vi "Replace Outside Typedef Control.vi"(6 "Dependent VIs":path[](array[path]), 8 "error in (no error)":errorcluster, 9 "Shared directory":path, 10 "Non-Library VI[]":string[](array[string]), 11 "Measurement Directory":path) -> (0 "error out":errorcluster)   [LabVIEW 2021, in "Multiple Converter.lvlib"]
uses:
  Multiple Converter.lvlib
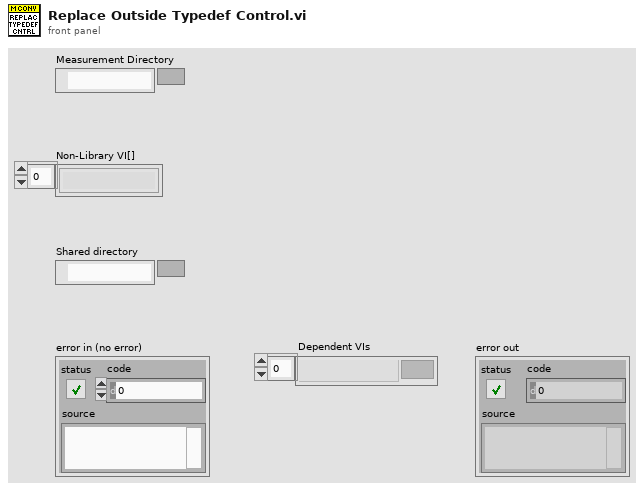
[diagram p1: front panel]
types:
  T1 = enum32{"not a typedef", "typedef", "strict typedef", "class private data"}
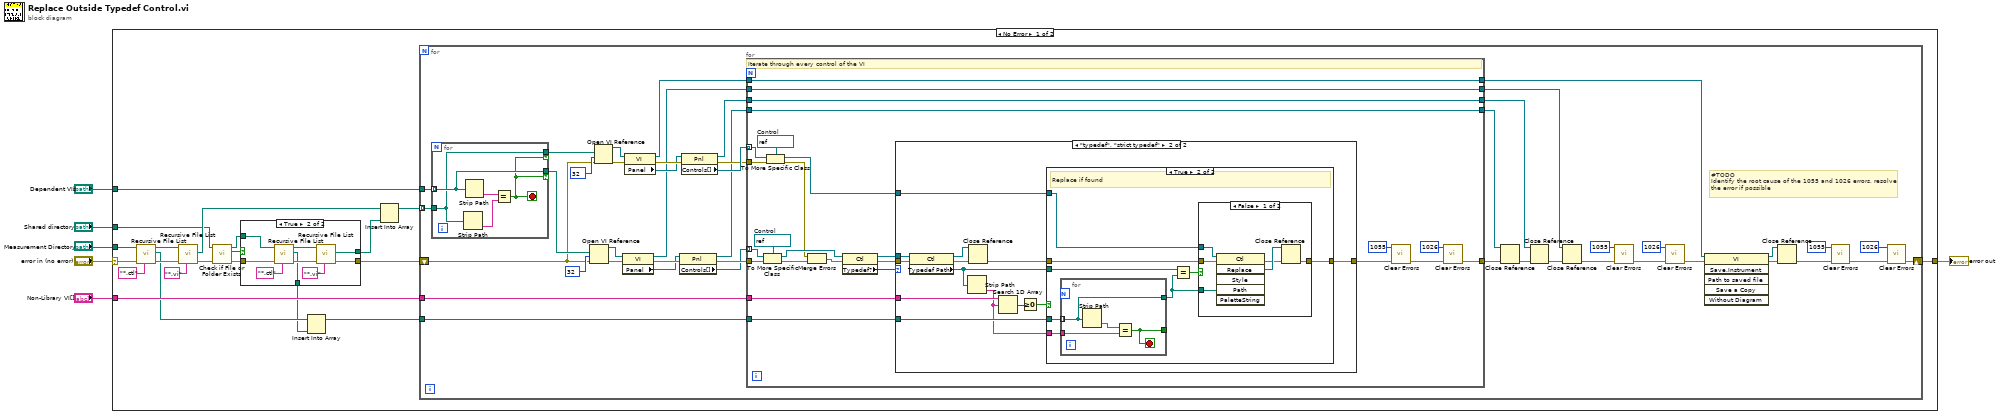
[diagram p0: block diagram]
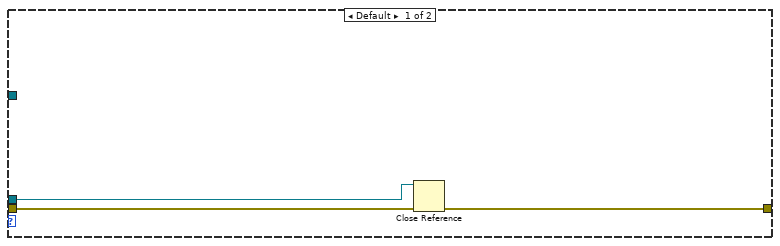
[diagram p2: hidden frame]
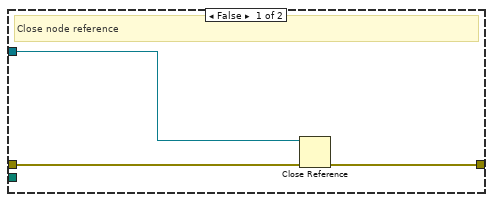
[diagram p3: hidden frame]
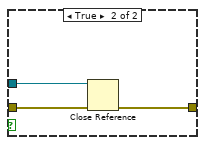
[diagram p4: hidden frame]
diagram:
  n1 = case shown="No Error" "error in (no error)" {
    selector: "error in (no error)" -> [w26 w152]
    tunnel: "Non-Library VI[]" -> [w27 _]
    tunnel: [w24 w152] -> w4
    tunnel: "Measurement Directory" -> [w22 _]
    tunnel: "Shared directory" -> [w8 _]
    tunnel: "Dependent VIs" -> [w7 _]
    frame No Error {
      n2 = call <vilib>:"Recursive File List.vi"("pattern"="*.ctl", "error in (no error)"=w26, "Folder Path"=w22) -> ("error out"=w23:errorcluster, "All Files in Dir"=w19:path[], "dup Folder Path"=w21:path)  [unwired: 4 in, 2 out]
      n3 = call <vilib>:"Recursive File List.vi"("pattern"="*.vi", "error in (no error)"=w23, "Folder Path"=w21) -> ("error out"=w17:errorcluster, "All Files in Dir"=w16:path[])  [unwired: 4 in, 3 out]
      n4 = call <vilib>:"Check if File or Folder Exists.vi"("error in (no error)"=w17, "path"=w8) -> ("error out"=w11:errorcluster, "file or folder exists?"=w10:bool, "dup path"=w9:path)  [unwired: 7 in]
      n5 = case shown="True" w10 {
        tunnel: [w142 w147] -> w18
        tunnel: w11 -> [w142 w146]
        tunnel: [_ w145] -> w13
        tunnel: [_ w144] -> w12
        tunnel: w9 -> [_ w143]
        frame False {
        }
        frame True {
          n6 = call <vilib>:"Recursive File List.vi"("pattern"="*.ctl", "error in (no error)"=w146, "Folder Path"=w143) -> ("error out"=w149:errorcluster, "All Files in Dir"=w145:path[], "dup Folder Path"=w150:path)  [unwired: 4 in, 2 out]
          n7 = call <vilib>:"Recursive File List.vi"("pattern"="*.vi", "error in (no error)"=w149, "Folder Path"=w150) -> ("error out"=w147:errorcluster, "All Files in Dir"=w144:path[])  [unwired: 4 in, 3 out]
        }
      }
      n8 = Insert Into Array(array=w19, new element=w13) -> (w14:path[])  [unwired: 1 in]
      n9 = Insert Into Array(array=w16, new element=w12) -> (w15:path[])  [unwired: 1 in]
      n10 = for {
        tunnel: w14 -> [w71]
        tunnel: w27 -> [w70]
        tunnel: w15 -> [w64] mode=indexing
        shift-right: [w37] -> w24
        shift-left: w18 -> [w61]
        tunnel: w7 -> [w65]
        # "#TODO\nIdentify the root cause of the 1055 and 1026 errors, resolve \nthe error if possible"
        n11 = for {
          tunnel: w65 -> [w139] mode=indexing
          tunnel: w64 -> [w138]
          tunnel: [w139] -> w63 if=w137
          tunnel: [w138] -> w60 if=w137
          stop <- w137 stop-if-true
          n12 = Strip Path(path=w138) -> (name=w140:string)  [unwired: 1 out]
          n13 = Strip Path(path=w139) -> (name=w141:string)  [unwired: 1 out]
          n14 = Equal?(x=w141, y=w140) -> (x = y?=w137:bool)
        }
        n15 = Open VI Reference(vi path=w63, options=32, error in (no error)=w61) -> (vi reference=w48:refnum<vi>, error out=w49:errorcluster)  [unwired: 3 in]
        n16 = Open VI Reference(vi path=w60, options=32, error in (no error)=w61) -> (vi reference=w56:refnum<vi>, error out=w50:errorcluster)  [unwired: 3 in]
        n17 = property class="VI"(reference=w48, error in=w49) -> (reference out=w31:refnum<vi>, error out=w51:errorcluster, "Panel"=w46:refnum<vi>)
        n18 = property class="VI"(reference=w56, error in=w50) -> (reference out=w55:refnum<vi>, error out=w54:errorcluster, "Panel"=w47:refnum<vi>)
        n19 = property class="Pnl"(reference=w46, error in=w51) -> (reference out=w28:refnum<vi>, error out=w45:errorcluster, "Controls[]"=w29:refnum<vi>[])
        n20 = property class="Pnl"(reference=w47, error in=w54) -> (reference out=w30:refnum<vi>, error out=w52:errorcluster, "Controls[]"=w53:refnum<vi>[])
        n21 = for {
          tunnel: w29 -> [w96] mode=indexing
          tunnel: w70 -> [w93]
          tunnel: w71 -> [w95]
          tunnel: w52 -> [w90]
          tunnel: w53 -> [w89] mode=indexing
          tunnel: w55 -> [w83]
          tunnel: w31 -> [w84]
          tunnel: [w83] -> w59
          tunnel: [w84] -> w57
          tunnel: w30 -> [w79]
          tunnel: w28 -> [w78]
          tunnel: [w79] -> w41
          tunnel: [w78] -> w40
          tunnel: w45 -> [w77]
          tunnel: [w73] -> w44
          w91 = refnum<vi> refnum  # Control
          w94 = refnum<vi> refnum  # Control
          # "Iterate through every control of the VI"
          n22 = To More Specific Class(target class=w94, reference=w96, error in=w77) -> (specific class reference=w92:refnum<vi>, error out=w86:errorcluster)
          n23 = To More Specific Class(target class=w91, reference=w89, error in=w90) -> (specific class reference=w88:refnum<vi>, error out=w85:errorcluster)
          n24 = Merge Errors(w85, w86) -> (w87:errorcluster)
          n25 = property class="Ctl"(reference=w92, error in=w87) -> (reference out=w81:refnum<vi>, error out=w82:errorcluster, "Typedef?"=w80:T1)
          n26 = case shown="\"typedef\", \"strict typedef\"" w80 {
            tunnel: w82 -> [w99 w101]
            tunnel: w81 -> [w97 w107]
            tunnel: [w98 w111] -> w76
            tunnel: w95 -> [_ w109]
            tunnel: w93 -> [_ w108]
            tunnel: w88 -> [_ w102]
            frame Default {
              n27 = Close Reference(reference=w97, error in (no error)=w99) -> (error out=w98:errorcluster)
            }
            frame "typedef", "strict typedef" {
              n28 = property class="Ctl"(reference=w107, error in=w101) -> (reference out=w103:refnum<vi>, error out=w104:errorcluster, "Typedef Path"=w105:path)
              n29 = Strip Path(path=w105) -> (name=w106:string)  [unwired: 1 out]
              n30 = Close Reference(reference=w103, error in (no error)=w104) -> (error out=w100:errorcluster)
              n31 = Search 1D Array(1D array=w108, element=w106) -> (index of element=w112:i32)  [unwired: 1 in]
              n32 = Greater Or Equal To 0?(x=w112) -> (x >= 0?=w110:bool)
              n33 = case shown="True" w110 {
                tunnel: [w115 w121] -> w111
                tunnel: w109 -> [_ w123]
                tunnel: w106 -> [_ w122]
                tunnel: w105 -> [_ w120]
                tunnel: w102 -> [w114 w117]
                tunnel: w100 -> [w113 w116]
                frame False {
                  # "Close node reference"
                  n34 = Close Reference(reference=w114, error in (no error)=w113) -> (error out=w115:errorcluster)
                }
                frame True {
                  # "Replace if found"
                  n35 = for {
                    tunnel: w123 -> [w134] mode=indexing
                    tunnel: w122 -> [w135]
                    tunnel: [w134] -> w119
                    tunnel: [w133] -> _
                    stop <- w133 stop-if-true
                    n36 = Strip Path(path=w134) -> (name=w136:string)  [unwired: 1 out]
                    n37 = Equal?(x=w136, y=w135) -> (x = y?=w133:bool)
                  }
                  n38 = Equal?(x=w120, y=w119) -> (x = y?=w118:bool)
                  n39 = case shown="False" w118 {
                    tunnel: w116 -> [w129 w132]
                    tunnel: [w127 w131] -> w121
                    tunnel: w119 -> [w126 _]
                    tunnel: w117 -> [w124 w130]
                    frame False {
                      n40 = invoke class="Ctl" method="Replace"(reference=w124, error in=w129, "Path"=w126) -> (error out=w125:errorcluster, "Replace"=w128:refnum<vi>)  [unwired: 3 in, 4 out]
                      n41 = Close Reference(reference=w128, error in (no error)=w125) -> (error out=w127:errorcluster)
                    }
                    frame True {
                      n42 = Close Reference(reference=w130, error in (no error)=w132) -> (error out=w131:errorcluster)
                    }
                  }
                }
              }
            }
          }
          n43 = call <vilib>:"Clear Errors.vi"("error in (no error)"=w76, "specific error code to clear (0: all)"=1055) -> ("error out"=w75:errorcluster)  [unwired: 4 in, 1 out]
          n44 = call <vilib>:"Clear Errors.vi"("error in (no error)"=w75, "specific error code to clear (0: all)"=1026) -> ("error out"=w73:errorcluster)  [unwired: 4 in, 1 out]
        }
        n45 = Close Reference(reference=w40, error in (no error)=w44) -> (error out=w43:errorcluster)
        n46 = Close Reference(reference=w41, error in (no error)=w43) -> (error out=w42:errorcluster)
        n47 = Close Reference(reference=w57, error in (no error)=w42) -> (error out=w58:errorcluster)
        n48 = call <vilib>:"Clear Errors.vi"("error in (no error)"=w58, "specific error code to clear (0: all)"=1055) -> ("error out"=w35:errorcluster)  [unwired: 4 in, 1 out]
        n49 = call <vilib>:"Clear Errors.vi"("error in (no error)"=w35, "specific error code to clear (0: all)"=1026) -> ("error out"=w39:errorcluster)  [unwired: 4 in, 1 out]
        n50 = invoke class="VI" method="Save.Instrument"(reference=w59, error in=w39) -> (reference out=w67:refnum<vi>, error out=w68:errorcluster)  [unwired: 4 in, 4 out]
        n51 = Close Reference(reference=w67, error in (no error)=w68) -> (error out=w69:errorcluster)
        n52 = call <vilib>:"Clear Errors.vi"("error in (no error)"=w69, "specific error code to clear (0: all)"=1055) -> ("error out"=w33:errorcluster)  [unwired: 4 in, 1 out]
        n53 = call <vilib>:"Clear Errors.vi"("error in (no error)"=w33, "specific error code to clear (0: all)"=1026) -> ("error out"=w37:errorcluster)  [unwired: 4 in, 1 out]
      }
    }
    frame Error {
    }
  }
  "error out" <- w4
